vi "Find Yellow2.vi"(6 "error in":errorcluster, 9 "SS File Path":path=path "C:/PokerSS/SS.png") -> (0 "error out":errorcluster)   [LabVIEW 2015]
uses:
  <vilib>/vision/NI_Vision_Development_Module.lvlib
panel:
  in  "File Path for Template":path=path "C:/Users/Bob Dabalina/Documents/Labview/Poker Hand2/YellowTemplate1.png"
  out "Image Out":T1(plugin-control)
  out "Matches (Find Yellow)":T2(array[cluster]) {"Bounding Box"."y" format="%.2f"; "Bounding Box"."x" format="%.2f"; "Position"."y" format="%.2f"; "Position"."x" format="%.2f"; "Score" format="%.2f"; "Scale" format="%.2f"; "Angle" format="%.2f"}
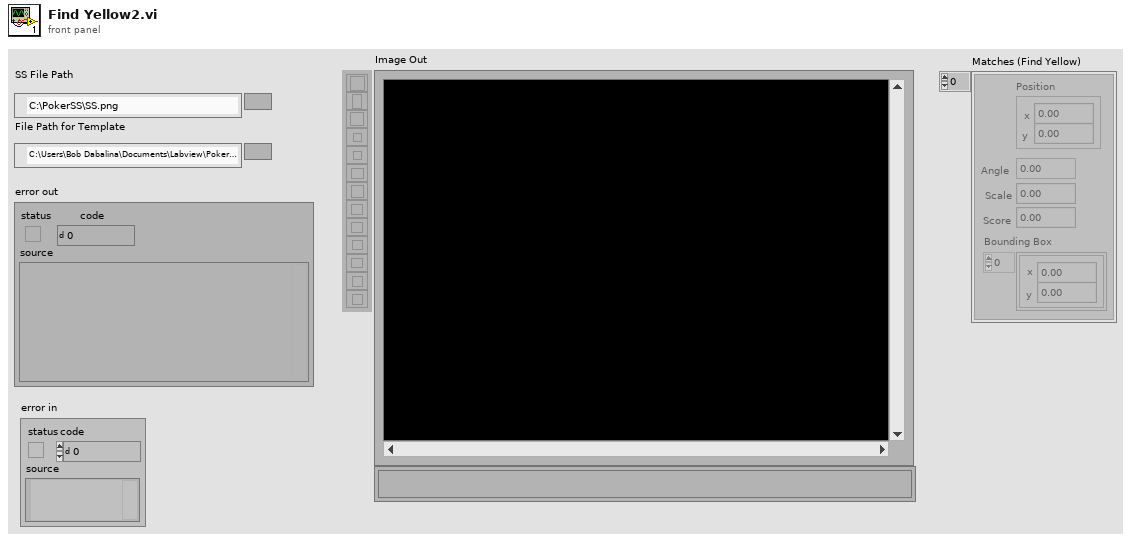
[diagram p1: front panel]
types:
  T1 = typedef "IMAQ Image.ctl" = refnum<image>
  T2 = cluster{"Position":cluster{"x":sgl, "y":sgl}, "Angle":sgl, "Scale":sgl, "Score":sgl, "Bounding Box":cluster{"x":sgl, "y":sgl}[]}[]
  T3 = typedef "Image Type" = u32
  T4 = cluster{"Position":cluster{"x":sgl, "y":sgl}, "Angle":sgl, "Scale":sgl, "Score":sgl, "Bounding Box":cluster{"x":sgl, "y":sgl}[]}
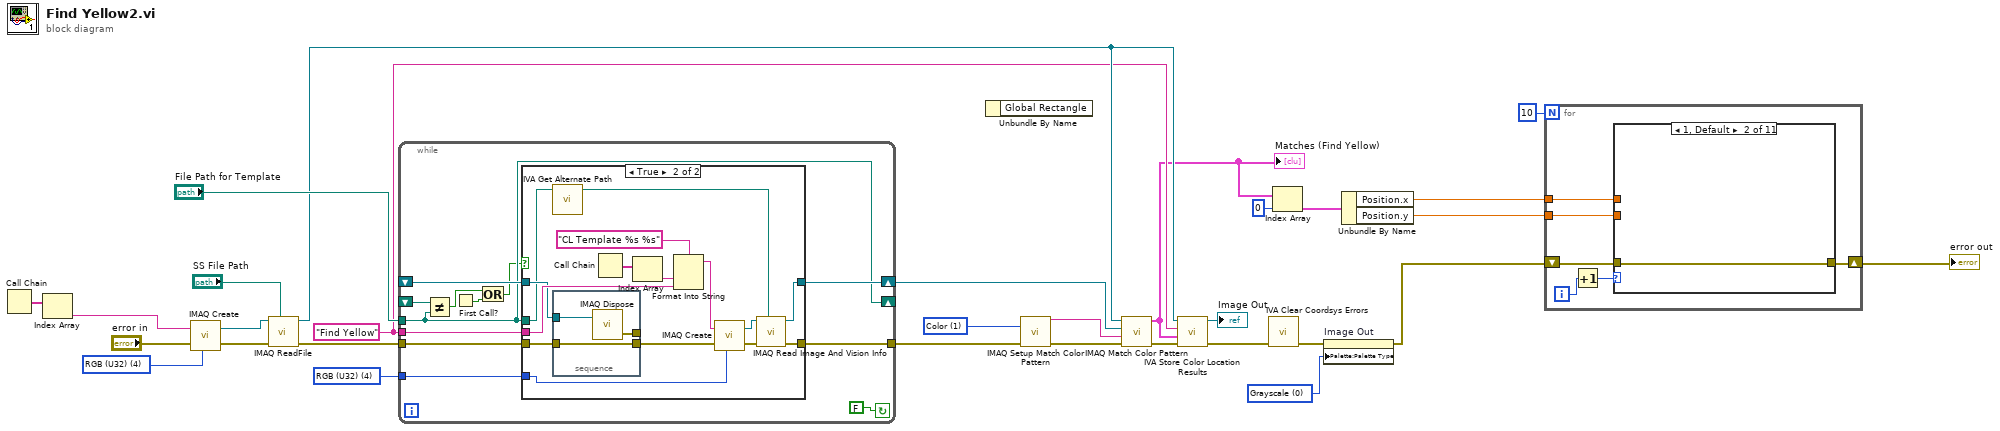
[diagram p0: block diagram]
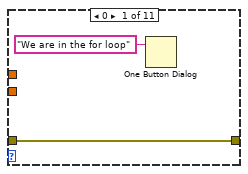
[diagram p2: hidden frame]
diagram:
  w10 = u32 0 items=["Grayscale", "Binary", "Gradient", "Rainbow", "Temperature", "User Defined", "Binary 16 Bit", "Gradient 16 Bit", "Rainbow 16 Bit", "Temperature 16 Bit", "User Defined 16 Bit"] ("Palette Type")
  w18 = "Find Yellow" ("Step Name")
  w21 = T3 4 items=["Grayscale (U8)", "Grayscale (I16)", "Grayscale (SGL)", "Complex (CSG)", "RGB (U32)", "HSL (U32)", "RGB (U64)"] ("Image Type")
  w23 = u32 1 items=["Color and Shape", "Color", "Shape"] ("Match Feature Mode")
  w24 = T3 4 items=["Grayscale (U8)", "Grayscale (I16)", "Grayscale (SGL)", "Complex (CSG)", "RGB (U32)", "HSL (U32)", "RGB (U64)", "Grayscale (U16)"] ("Image Type")
  n1 = Call Chain() -> (call chain=w26:string[])
  n2 = Index Array(array=w26) -> (element=w25:string)  [unwired: 1 in]
  n3 = call "IMAQ Create"("Image Name"=w25, "Image Type"=w24, "error in (no error)"="error in") -> ("New Image"=w29:T1, "error out"=w28:errorcluster)  [unwired: 1 in, 1 out]
  n4 = call "IMAQ ReadFile"("File Path"="SS File Path", "error in (no error)"=w28, "Image"=w29) -> ("error out"=w30:errorcluster, "Image Out"=w19:T1)  [unwired: 2 in, 5 out]
  n5 = while {
    shift-right: [w42] -> w15
    shift-left: _ -> [w41]
    tunnel: [w39] -> w14
    tunnel: w30 -> [w38]
    tunnel: "File Path for Template" -> [w34]
    tunnel: w21 -> [w37]
    tunnel: w18 -> [w36]
    shift-right: [w34] -> _
    shift-left: _ -> [w35]
    stop <- FALSE continue-if-true
    n6 = Not Equal?(x=w35, y=w34) -> (x != y?=w32:bool)
    n7 = First Call?() -> (First Call?: T/F=w33:bool)
    n8 = Or(x=w32, y=w33) -> (x .or. y?=w31:bool)
    n9 = case shown="True" w31 {
      tunnel: [w44 w57] -> w42
      tunnel: w41 -> [w44 w49]
      tunnel: [w43 w54] -> w39
      tunnel: w38 -> [w43 w48]
      tunnel: w37 -> [_ w53]
      tunnel: w36 -> [_ w50]
      tunnel: w34 -> [_ w46]
      frame False {
      }
      frame True {
        n10 = call <vilib>:"IVA Get Alternate Path.vi"("Path In"=w46) -> ("Path Out"=w45:path)  [unwired: 10 out]
        n11 = stacked-sequence {
          tunnel: w49 -> [w62]
          tunnel: w48 -> [w61]
          tunnel: [w61] -> w47
          tunnel: [w60] -> _
          frame #0 {
            n12 = call "IMAQ Dispose"("Image"=w62) -> ("error out"=w60:errorcluster)  [unwired: 2 in, 3 out]
          }
        }
        n13 = Call Chain() -> (call chain=w52:string[])
        n14 = Index Array(array=w52) -> (element=w51:string)  [unwired: 1 in]
        n15 = Format Into String(format string="CL Template %s %s" ("Image Name"), w51, w50) -> (resulting string=w59:string)  [unwired: 2 in, 1 out]
        n16 = call "IMAQ Create"("Image Name"=w59, "Image Type"=w53, "error in (no error)"=w47) -> ("New Image"=w56:T1, "error out"=w55:errorcluster)  [unwired: 1 in, 1 out]
        n17 = call "IMAQ Read Image And Vision Info"("File Path"=w45, "error in (no error)"=w55, "Image"=w56) -> ("error out"=w54:errorcluster, "Image Out"=w57:T1)  [unwired: 1 in, 6 out]
      }
    }
  }
  n18 = Unbundle By Name() -> ()  [unwired: 1 in, 1 out]
  n19 = call "IMAQ Setup Match Color Pattern"("Match Feature Mode"=w23, "error in (no error)"=w14) -> ("Match Color Pattern Setup Data"=w17:string, "error out"=w16:errorcluster)  [unwired: 7 in, 5 out]
  n20 = call "IMAQ Match Color Pattern"("error in (no error)"=w16, "Match Color Pattern Setup Data"=w17, "Template Image"=w15, "Image"=w19) -> ("error out"=w20:errorcluster, "Matches"=w8:T2)  [unwired: 3 in, 3 out]
  "Matches (Find Yellow)" <- w8
  n21 = call <vilib>:"IVA Store Color Location Results.vi"("error in (no error)"=w20, "Matches"=w8, "Step Name"=w18, "Image in"=w19) -> ("error out"=w13:errorcluster, "Image dup"=→"Image Out":T1)  [unwired: 6 out]
  n22 = call <vilib>:"IVA Clear Coordsys Errors.vi"("error in (no error)"=w13) -> ("error out"=w12:errorcluster)  [unwired: 10 in]
  n23 = Index Array(array=w8, index=0) -> (element=w6:T4)
  n24 = property on="Image Out" class="ImageControl"(error in=w12, "Palette:Palette Type"=w10) -> (error out=w2:errorcluster)  [unwired: 1 in, 1 out]
  n25 = Unbundle By Name(w6) -> ("Position.x"=w4:sgl, "Position.y"=w3:sgl)
  n26 = for {
    N: 10 -> [_]
    tunnel: w4 -> [w67]
    tunnel: w3 -> [w66]
    shift-right: [w65] -> w1
    shift-left: w2 -> [w64]
    i -> [w68]
    n27 = Increment(x=w68) -> (x+1=w63:i32)
    n28 = case shown="1, Default" w63 {
      tunnel: w67 -> [_ _ _ _ _ _ _ _ _ _ _]
      tunnel: w66 -> [_ _ _ _ _ _ _ _ _ _ _]
      tunnel: [w70 w71 w72 w73 w74 w75 w76 w77 w78 w79 w80] -> w65
      tunnel: w64 -> [w70 w71 w72 w73 w74 w75 w76 w77 w78 w79 w80]
      frame 0 {
        n29 = One Button Dialog(message="We are in the for loop") -> ()  [unwired: 1 in, 1 out]
      }
      frame 1, Default {
      }
      frame 2 {
      }
      frame 3 {
      }
      frame 4 {
      }
      frame 5 {
      }
      frame 6 {
      }
      frame 7 {
      }
      frame 8 {
      }
      frame 9 {
      }
      frame 10 {
      }
    }
  }
  "error out" <- w1
